vi "Get Events.vi"(0 "Display State In":T2, 9 "Container State":T6, 11 "error in (no error)":errorcluster) -> (4 "Display State Out":T2, 8 "Events":T1, 15 "error out":errorcluster)   [LabVIEW 2020, in "KTable.xctl"]
uses:
  KTable.xctl
  <vilib>/_xctls/Container State.ctl
  <vilib>/_xctls/XControlSupport.lvlib
  ColumnType.ctl
  ColumnSpec.ctl
  State.ctl
  Event Type.ctl
  Event Data.ctl
  Table Properties.ctl
  Events.ctl
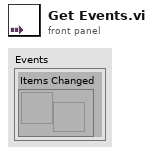
[diagram p1: front panel]
types:
  T1 = typedef "KTable.xctl/Events.ctl" = cluster{"Items Changed":refnum<user-event>}
  T2 = typedef "KTable.xctl/State.ctl" = cluster{"Columns":T3[], "Listbox":refnum<vi>, "Default row":string[], "Properties":T5, "Events":T1, "Locked":bool[][], "Size":cluster{"Rows":i32, "Columns":i32}, "rings":i32[][], "DefColors":u32[], "highlight row":bool}
  T3 = typedef "KTable.xctl/ColumnSpec.ctl" = cluster{"Name":string, "Type":T4, "Width":i32, "Strings":string[], "Position":enum16{"Left", "Center", "Right"}, "locked":bool, "cds":cluster{"Strings":string[]}[][], "Hide NaN":bool}
  T4 = typedef "KTable.xctl/ColumnType.ctl" = enum16{"String", "Enum", "Int", "Double", "Boolean", "Ring", "Formula", "Color"}
  T5 = typedef "KTable.xctl/Table Properties.ctl" = cluster{"Vertical scrollbar":bool, "User add/delete":bool, "Max rows":i32, "Row headers":bool}
  T6 = typedef "XControlSupport.lvlib/Container State.ctl" = cluster{"Indicator?":bool, "Run Mode?":bool, " Refnum":refnum<vi>}
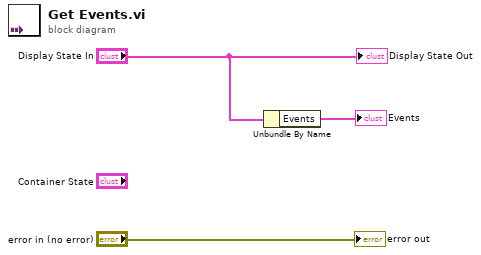
[diagram p0: block diagram]
diagram:
  n1 = Unbundle By Name("Display State In") -> ("Events"=→"Events":T1)
  "Display State Out" <- "Display State In"
  "error out" <- "error in (no error)"
